vi "Group_Project-REV4.vi"() -> ()   [LabVIEW 2022 SP3]
uses:
  Control 1.ctl
panel:
  out "Train 0s":bool
  out "Speed up train?":string
  out "Train 65%":bool
  out "Train 35%":bool
  out "How long has train departed (ms)":dbl
  out "Numeric 6":u32
  out "Total wait time (ms)":dbl
  out "One sensor detected?":bool=TRUE
  out "Refresh timer with less traffic (ms)":dbl
  out "TIme add up (ms)":dbl
  in  "Sensor Traffic 2":bool
  in  "Sensor Traffic 1":bool
  out "Traffic light, Red-Amber-Green":bool[](array[boolean])
  out "Busy traffic?":bool
  out "Boom gate":string
  in  "Sensor Train 2":bool
  in  "Sensor Train 1":bool
  out "Train go which way":dbl
  out "Numeric 5":u32
  out "RED LIGHT":bool
  out "Numeric 4":u32
  out "GREEN LIGHT":bool
  out "Train?":bool
  out "Numeric 3":u32
  out "Vehicle detected":i32
  out "Station light":bool
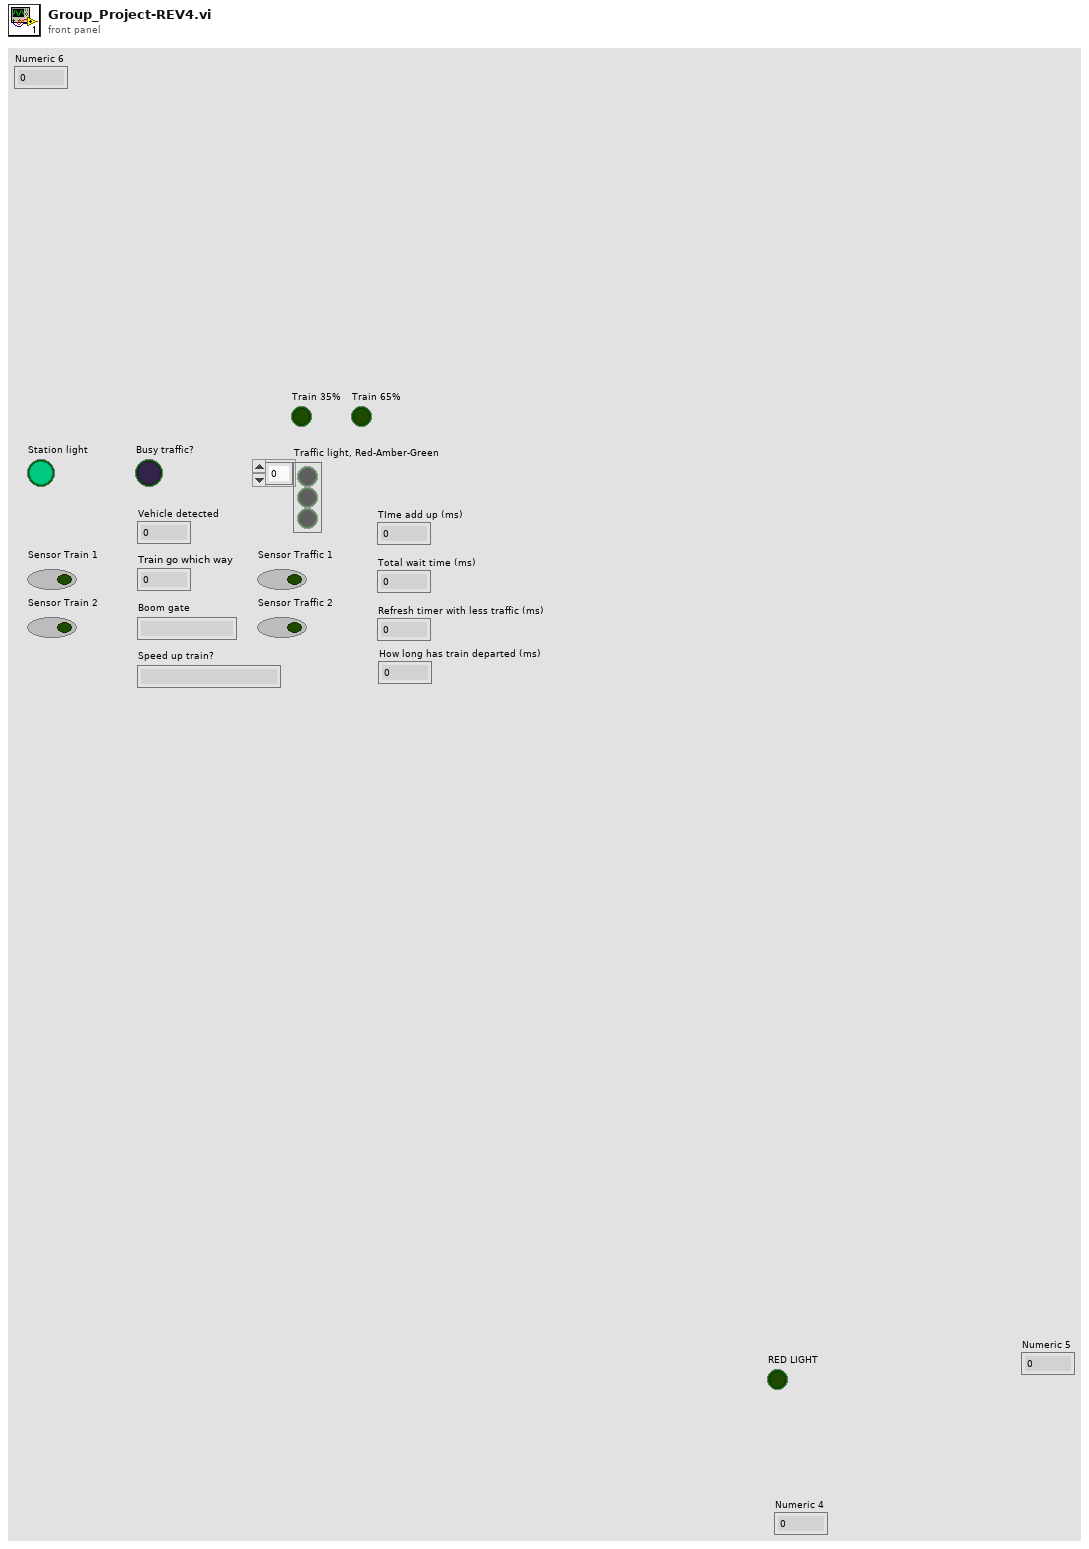
[diagram p1: front panel]
types:
  T1 = typedef "Control 1.ctl" = enum16{"None", "Down", "Up"}
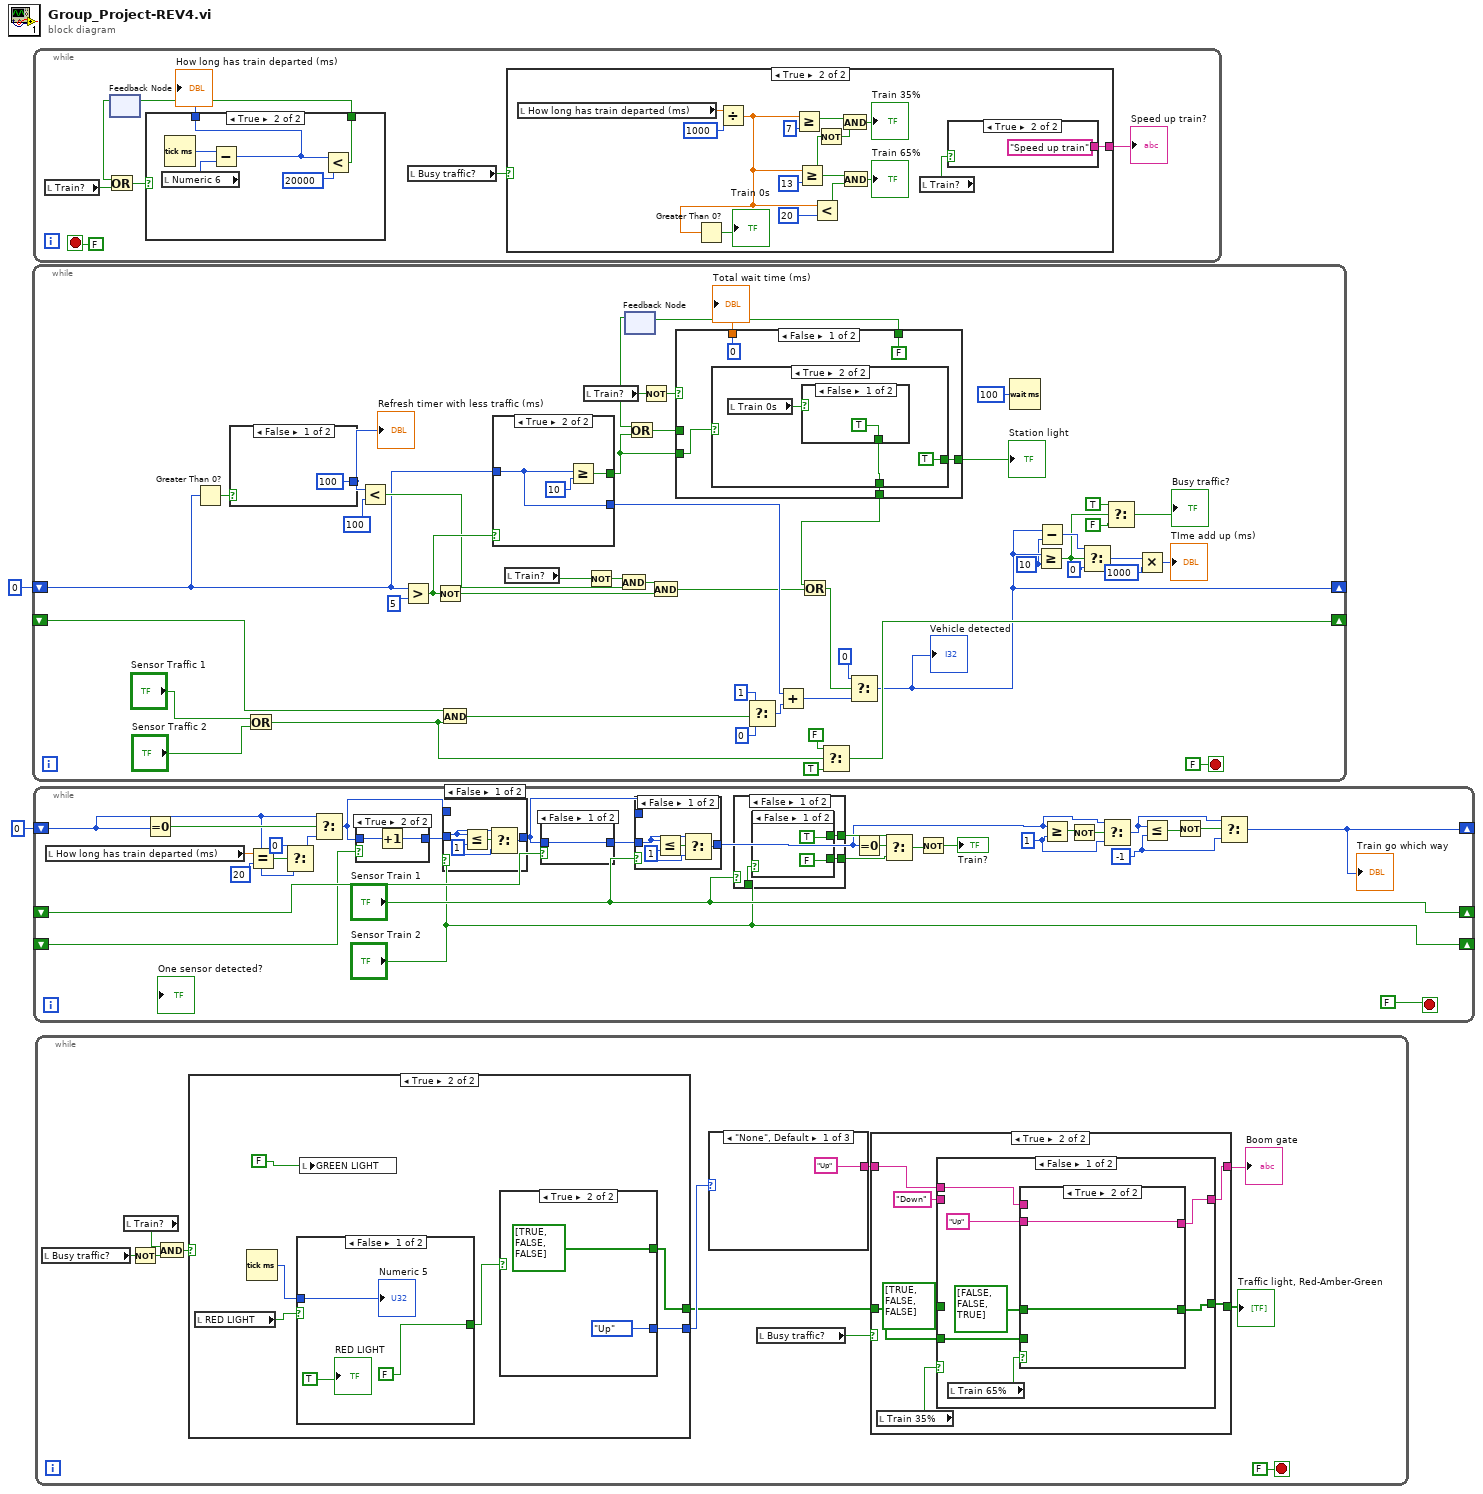
[diagram p0: block diagram]
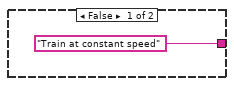
[diagram p2: hidden frame]
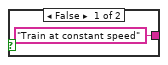
[diagram p3: hidden frame]
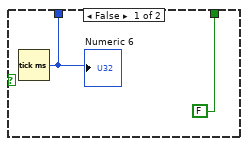
[diagram p4: hidden frame]
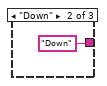
[diagram p8: hidden frame]
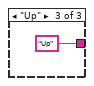
[diagram p9: hidden frame]
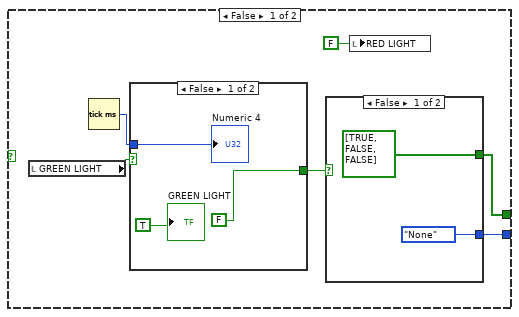
[diagram p10: hidden frame]
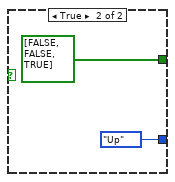
[diagram p11: hidden frame]
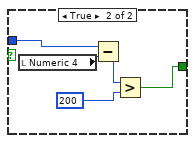
[diagram p12: hidden frame]
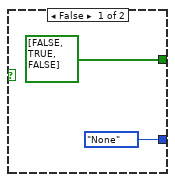
[diagram p13: hidden frame]
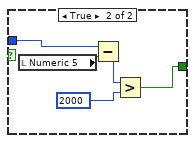
[diagram p14: hidden frame]
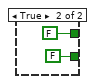
[diagram p15: hidden frame]
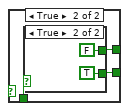
[diagram p16: hidden frame]
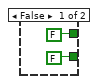
[diagram p17: hidden frame]
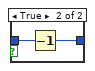
[diagram p19: hidden frame]
diagram:
  n1 = while {
    shift-right: [w37] -> _
    shift-left: 0 -> [w10]
    shift-right: [w41] -> _
    shift-left: _ -> [w40]
    stop <- FALSE stop-if-true
    w36 = 10
    n2 = Greater Than 0?(x=w10) -> (x > 0?=w9:bool)
    n3 = case shown="False" w9 {
      tunnel: [100 w81] -> w31
      frame False {
      }
      frame True {
        n4 = Tick Count (ms)() -> (millisecond timer value=w82:u32)
        n5 = Quotient & Remainder(x=w82, y=10000) -> (x-y*floor(x/y)=w81:u32)  [unwired: 1 out]
      }
    }
    "Refresh timer with less traffic (ms)" <- w31
    n6 = Or(x="Sensor Traffic 1", y="Sensor Traffic 2") -> (x .or. y?=w23:bool)
    n7 = Less?(x=w31, y=100) -> (x < y?=w13:bool)
    n8 = Greater?(x=w10, y=5) -> (0:w19:bool)
    n9 = Not(x=w19) -> (.not. x?=w22:bool)
    n10 = And(x=w40, y=w23) -> (x .and. y?=w51:bool)
    n11 = case shown="True" w19 {
      tunnel: w10 -> [w84 w86]
      tunnel: [w84 w86] -> w43
      tunnel: [FALSE w85] -> w3
      frame False {
      }
      frame True {
        n12 = Greater Or Equal?(x=w86, y=10) -> (x >= y?=w85:bool)
      }
    }
    n13 = local read "Train?"() -> (w11:bool)
    n14 = local read "Train?"() -> (w4:bool)
    n15 = Not(x=w11) -> (.not. x?=w12:bool)
    n16 = And(x=w12, y=w13) -> (x .and. y?=w14:bool)
    n17 = feedback #1() -> (w20:bool)  [unwired: 1 in]
    n18 = Or(x=w20, y=w3) -> (x .or. y?=w6:bool)
    n19 = Not(x=w4) -> (.not. x?=w5:bool)
    n20 = And(x=w14, y=w22) -> (x .and. y?=w18:bool)
    n21 = case shown="False" w5 {
      tunnel: w6 -> [_ w67]
      tunnel: [w54 w66] -> w42
      tunnel: [FALSE w65] -> w16
      tunnel: [w53 w64] -> w15
      tunnel: [0 w63] -> w8
      tunnel: w3 -> [w52 _]
      frame False {
        n22 = case shown="True" w52 {
          tunnel: [w57 TRUE] -> w54
          tunnel: [w57 w58] -> w53
          frame False {
            w57 = FALSE
          }
          frame True {
            n23 = local read "Train 0s"() -> (w59:bool)
            n24 = case shown="False" w59 {
              tunnel: [TRUE FALSE] -> w58
              frame False {
              }
              frame True {
              }
            }
          }
        }
      }
      frame True {
        n25 = case shown="True" w67 {
          tunnel: [w68 w73] -> w65
          tunnel: [w68 TRUE] -> w66
          tunnel: [w69 w71] -> w63
          tunnel: [w68 w72] -> w64
          frame False {
            w68 = FALSE
            n26 = Tick Count (ms)() -> (millisecond timer value=w69:u32)
            "Numeric 3" <- w69
          }
          frame True {
            w70 = 10000
            n27 = local read "Numeric 3"() -> (w78:u32)
            n28 = local read "TIme add up (ms)"() -> (w74:dbl)
            n29 = Tick Count (ms)() -> (millisecond timer value=w76:u32)
            n30 = Subtract(x=w76, y=w78) -> (x-y=w75:u32)
            n31 = Subtract(x=w75, y=w74) -> (x-y=w71:dbl)
            n32 = Greater Or Equal?(x=w71, y=w70) -> (x >= y?=w72:bool)
            n33 = Less?(x=w71, y=w70) -> (x < y?=w73:bool)
          }
        }
      }
    }
    "Station light" <- w42
    "Total wait time (ms)" <- w8
    n34 = feedback-in #1(w16) -> ()
    n35 = Select(t=1, s=w51, f=0) -> (s? t:f=w50:i32)
    n36 = Add(x=w43, y=w50) -> (x+y=w46:i32)
    n37 = Or(x=w15, y=w18) -> (x .or. y?=w17:bool)
    n38 = Select(t=FALSE, s=w23, f=TRUE) -> (s? t:f=w41:bool)
    n39 = Select(t=0, s=w17, f=w46) -> (s? t:f=w37:i32)
    "Vehicle detected" <- w37
    n40 = Wait (ms)(milliseconds to wait=100) -> ()  [unwired: 1 out]
    n41 = Greater Or Equal?(x=w37, y=w36) -> (x >= y?=w30:bool)
    n42 = Subtract(x=w37, y=w36) -> (x-y=w35:i32)
    n43 = Select(t=w35, s=w30, f=0) -> (s? t:f=w34:i32)
    n44 = Select(t=TRUE, s=w30, f=FALSE) -> (s? t:f=→"Busy traffic?":bool)
    n45 = Multiply(x=w34, y=1000) -> (x*y=→"TIme add up (ms)":i32)
  }
  n46 = while {
    stop <- FALSE stop-if-true
    n47 = local read "Train?"() -> (w88:bool)
    n48 = feedback #2() -> (w92:bool)  [unwired: 1 in]
    n49 = Or(x=w92, y=w88) -> (x .or. y?=w94:bool)
    n50 = case shown="True" w94 {
      tunnel: [FALSE w116] -> w93
      tunnel: [w115 w117] -> w91
      frame False {
        n51 = Tick Count (ms)() -> (millisecond timer value=w115:u32)
        "Numeric 6" <- w115
      }
      frame True {
        n52 = local read "Numeric 6"() -> (w120:u32)
        n53 = Tick Count (ms)() -> (millisecond timer value=w119:u32)
        n54 = Subtract(x=w119, y=w120) -> (x-y=w117:u32)
        n55 = Less?(x=w117, y=20000) -> (x < y?=w116:bool)
      }
    }
    "How long has train departed (ms)" <- w91
    n56 = feedback-in #2(w93) -> ()
    n57 = local read "Busy traffic?"() -> (w90:bool)
    n58 = case shown="True" w90 {
      tunnel: ["Train at constant speed" w107] -> w89
      frame False {
      }
      frame True {
        n59 = local read "How long has train departed (ms)"() -> (w111:dbl)
        n60 = Divide(x=w111, y=1000) -> (x/y=w98:dbl)
        n61 = Greater Than 0?(x=w98) -> (x > 0?=→"Train 0s":bool)
        n62 = Greater Or Equal?(x=w98, y=7) -> (x >= y?=w104:bool)
        n63 = Greater Or Equal?(x=w98, y=13) -> (x >= y?=w103:bool)
        n64 = Less?(x=w98, y=20) -> (x < y?=w99:bool)
        n65 = Not(x=w103) -> (.not. x?=w105:bool)
        n66 = And(x=w104, y=w105) -> (x .and. y?=→"Train 35%":bool)
        n67 = And(x=w103, y=w99) -> (x .and. y?=→"Train 65%":bool)
        n68 = local read "Train?"() -> (w100:bool)
        n69 = case shown="True" w100 {
          tunnel: ["Train at constant speed" "Speed up train"] -> w107
          frame False {
          }
          frame True {
          }
        }
      }
    }
    "Speed up train?" <- w89
  }
  n70 = while {
    shift-right: [w131] -> _
    shift-left: 0 -> [w121]
    shift-right: ["Sensor Train 2"] -> _
    shift-left: _ -> [w133]
    shift-right: ["Sensor Train 1"] -> _
    shift-left: _ -> [w134]
    stop <- FALSE stop-if-true
    w137 = -1
    w140 = 1
    n71 = local read "How long has train departed (ms)"() -> (w127:dbl)
    n72 = Equal To 0?(x=w121) -> (x = 0?=w124:bool)
    n73 = Equal?(x=w127, y=20) -> (x = y?=w126:bool)
    n74 = Select(t=0, s=w126, f=w121) -> (s? t:f=w123:i32)
    n75 = Select(t=w121, s=w124, f=w123) -> (s? t:f=w122:i32)
    n76 = case shown="True" w133 {
      tunnel: [w178 w180] -> w150
      tunnel: w122 -> [w178 w179]
      frame False {
      }
      frame True {
        n77 = Increment(x=w179) -> (x+1=w180:i32)
      }
    }
    n78 = case shown="False" "Sensor Train 2" {
      tunnel: w150 -> [w175 _]
      tunnel: [w173 w177] -> w149
      tunnel: w122 -> [_ w177]
      frame False {
        w174 = 1
        n79 = Less Or Equal?(x=w175, y=w174) -> (x <= y?=w176:bool)
        n80 = Select(t=w175, s=w176, f=w174) -> (s? t:f=w173:i32)
      }
      frame True {
      }
    }
    n81 = case shown="False" w134 {
      tunnel: w149 -> [w170 w172]
      tunnel: [w170 w171] -> w148
      frame False {
      }
      frame True {
        n82 = Decrement(x=w172) -> (x-1=w171:i32)
      }
    }
    n83 = case shown="False" "Sensor Train 1" {
      tunnel: w149 -> [_ w169]
      tunnel: w148 -> [w166 _]
      tunnel: [w165 w169] -> w141
      frame False {
        w167 = 1
        n84 = Less Or Equal?(x=w166, y=w167) -> (x <= y?=w168:bool)
        n85 = Select(t=w166, s=w168, f=w167) -> (s? t:f=w165:i32)
      }
      frame True {
      }
    }
    n86 = case shown="False" "Sensor Train 1" {
      tunnel: "Sensor Train 2" -> [w151 w160]
      tunnel: [w152 w158] -> w146
      tunnel: [w153 w159] -> w145
      frame False {
        n87 = case shown="False" w151 {
          tunnel: [TRUE FALSE] -> w152
          tunnel: [FALSE FALSE] -> w153
          frame False {
          }
          frame True {
          }
        }
      }
      frame True {
        n88 = case shown="True" w160 {
          tunnel: [FALSE FALSE] -> w158
          tunnel: [FALSE TRUE] -> w159
          frame False {
          }
          frame True {
          }
        }
      }
    }
    n89 = Equal To 0?(x=w141) -> (x = 0?=w147:bool)
    n90 = Select(t=w146, s=w147, f=w145) -> (s? t:f=w144:bool)
    n91 = Not(x=w144) -> (.not. x?=→"Train?":bool)
    n92 = Greater Or Equal?(x=w141, y=w140) -> (x >= y?=w142:bool)
    n93 = Not(x=w142) -> (.not. x?=w143:bool)
    n94 = Select(t=w141, s=w143, f=w140) -> (s? t:f=w136:i32)
    n95 = Less Or Equal?(x=w136, y=w137) -> (x <= y?=w139:bool)
    n96 = Not(x=w139) -> (.not. x?=w138:bool)
    n97 = Select(t=w136, s=w138, f=w137) -> (s? t:f=w131:i32)
    "Train go which way" <- w131
  }
  n98 = while {
    stop <- FALSE stop-if-true
    n99 = local read "Busy traffic?"() -> (w185:bool)
    n100 = local read "Train?"() -> (w182:bool)
    n101 = Not(x=w185) -> (.not. x?=w183:bool)
    n102 = And(x=w182, y=w183) -> (x .and. y?=w184:bool)
    n103 = case shown="True" w184 {
      tunnel: [w217 w236] -> w187
      tunnel: [w218 w237] -> w191
      frame False {
        n104 = local read "GREEN LIGHT"() -> (w222:bool)
        n105 = Tick Count (ms)() -> (millisecond timer value=w220:u32)
        n106 = case shown="False" w222 {
          tunnel: [FALSE w230] -> w221
          tunnel: w220 -> [w228 w234]
          frame False {
            "Numeric 4" <- w228
            "GREEN LIGHT" <- TRUE
          }
          frame True {
            n107 = local read "Numeric 4"() -> (w233:u32)
            n108 = Subtract(x=w234, y=w233) -> (x-y=w232:u32)
            n109 = Greater?(x=w232, y=200) -> (0:w230:bool)
          }
        }
        n110 = case shown="False" w221 {
          tunnel: [bool[] [TRUE, FALSE, FALSE] bool[] [FALSE, FALSE, TRUE]] -> w217
          tunnel: [Control_1."None" Control_1."Up"] -> w218
          frame False {
          }
          frame True {
          }
        }
        n111 = local write "RED LIGHT"(FALSE) -> ()
      }
      frame True {
        n112 = local read "RED LIGHT"() -> (w240:bool)
        n113 = Tick Count (ms)() -> (millisecond timer value=w239:u32)
        n114 = case shown="False" w240 {
          tunnel: [FALSE w248] -> w235
          tunnel: w239 -> [w246 w252]
          frame False {
            "Numeric 5" <- w246
            "RED LIGHT" <- TRUE
          }
          frame True {
            n115 = local read "Numeric 5"() -> (w251:u32)
            n116 = Subtract(x=w252, y=w251) -> (x-y=w250:u32)
            n117 = Greater?(x=w250, y=2000) -> (0:w248:bool)
          }
        }
        n118 = local write "GREEN LIGHT"(FALSE) -> ()
        n119 = case shown="True" w235 {
          tunnel: [bool[] [FALSE, TRUE, FALSE] bool[] [TRUE, FALSE, FALSE]] -> w236
          tunnel: [Control_1."None" Control_1."Up"] -> w237
          frame False {
          }
          frame True {
          }
        }
      }
    }
    n120 = case shown="\"None\", Default" w191 {
      tunnel: ["Up" "Down" "Up"] -> w189
      frame "None", Default {
      }
      frame "Down" {
      }
      frame "Up" {
      }
    }
    n121 = local read "Busy traffic?"() -> (w181:bool)
    n122 = case shown="True" w181 {
      tunnel: w189 -> [w193 w195]
      tunnel: [w193 w196] -> w188
      tunnel: w187 -> [w192 w194]
      tunnel: [w192 w197] -> w186
      frame False {
      }
      frame True {
        n123 = local read "Train 35%"() -> (w199:bool)
        n124 = case shown="False" w199 {
          tunnel: "Down" -> [_ w213]
          tunnel: [w205 w213] -> w196
          tunnel: bool[] [TRUE, FALSE, FALSE] -> [_ w212]
          tunnel: [w203 w212] -> w197
          tunnel: w195 -> [w202 _]
          tunnel: w194 -> [w201 _]
          frame False {
            n125 = local read "Train 65%"() -> (w207:bool)
            n126 = case shown="True" w207 {
              tunnel: [w209 w211] -> w205
              tunnel: [w208 w210] -> w203
              tunnel: "Up" -> [_ w211]
              tunnel: bool[] [FALSE, FALSE, TRUE] -> [_ w210]
              tunnel: w202 -> [w209 _]
              tunnel: w201 -> [w208 _]
              frame False {
              }
              frame True {
              }
            }
          }
          frame True {
          }
        }
      }
    }
    "Boom gate" <- w188
    "Traffic light, Red-Amber-Green" <- w186
  }
